vi "Update montage.vi"(4 "Frames info":T1, 6 "Frame's rel. index":i32=1 min=0, 8 "Error in":errorcluster, 9 "Single patch image":T2, 10 "Coordinates of montage positions":cluster{"Offset Left/Top":i32[]}[](array[cluster]), 11 "Image (Montage)":T2) -> (0 "error out":errorcluster, 3 "Image (Montage)":T2)   [LabVIEW 2020]
uses:
  <vilib>/vision/Image Controls.llb/IMAQ Image.ctl
  <vilib>/vision/NI_Vision_Development_Module.lvlib
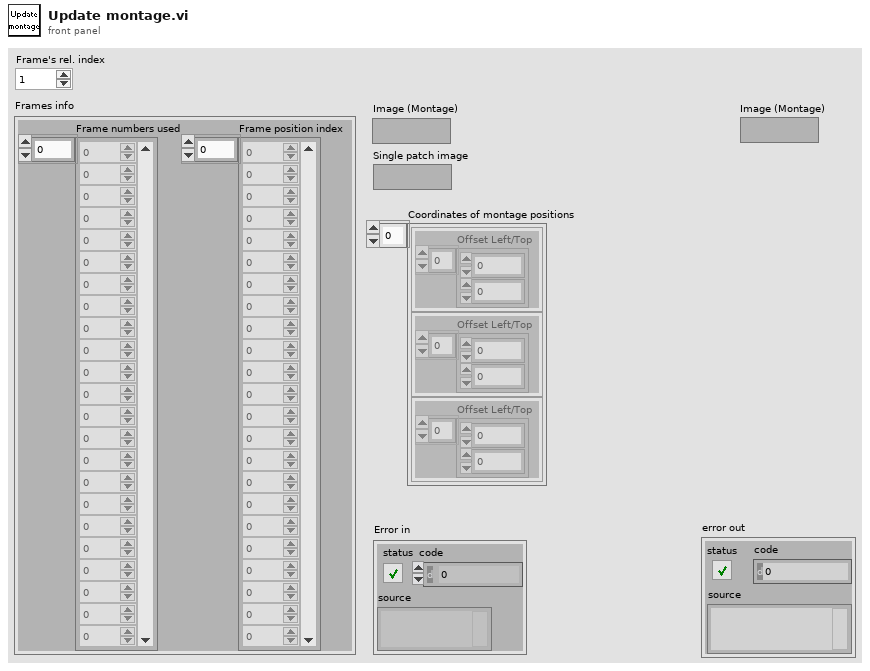
[diagram p1: front panel]
types:
  T1 = cluster{"Frame numbers used":i32[], "Frame position index":i32[]}
  T2 = typedef "IMAQ Image.ctl" = refnum<image>
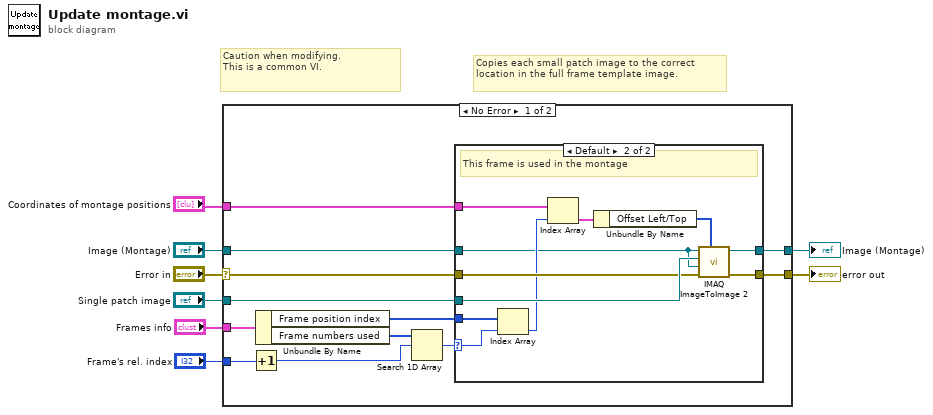
[diagram p0: block diagram]
diagram:
  # "Caution when modifying.\nThis is a common VI."
  # "Copies each small patch image to the correct location in the full frame template image."
  n1 = case shown="No Error" "Error in" {
    selector: "Error in" -> [w9 w35]
    tunnel: [w20 w34] -> w8
    tunnel: [w19 w35] -> w7
    tunnel: "Single patch image" -> [w18 _]
    tunnel: "Image (Montage)" -> [w17 w34]
    tunnel: "Coordinates of montage positions" -> [w16 _]
    tunnel: "Frames info" -> [w15 _]
    tunnel: "Frame's rel. index" -> [w14 _]
    frame No Error {
      n2 = Increment(x=w14) -> (x+1=w12:i32)
      n3 = Unbundle By Name(w15) -> ("Frame position index"=w11:i32[], "Frame numbers used"=w13:i32[])
      n4 = Search 1D Array(1D array=w13, element=w12) -> (index of element=w10:i32)  [unwired: 1 in]
      n5 = case shown="Default" w10 {
        selector: w10 -> [_ w24]
        tunnel: [w22 w33] -> w20
        tunnel: [w21 w31] -> w19
        tunnel: w18 -> [_ w30]
        tunnel: w17 -> [w22 w23]
        tunnel: w9 -> [w21 w29]
        tunnel: w16 -> [_ w28]
        tunnel: w11 -> [_ w26]
        frame -1 {
          # "This frame is not used in the montage"
        }
        frame Default {
          # "This frame is used in the montage"
          n6 = Index Array(array=w26, index=w24) -> (element=w25:i32)
          n7 = Index Array(array=w28, index=w25) -> (element=w27:cluster{"Offset Left/Top":i32[]})
          n8 = Unbundle By Name(w27) -> ("Offset Left/Top"=w32:i32[])
          n9 = call "IMAQ ImageToImage 2"("Offset Left/Top"=w32, "error in (no error)"=w29, "Image Dst"=w23, "Image Src (Small)"=w30, "Image Src (Large)"=w23) -> ("error out"=w31:errorcluster, "Image Dst Out"=w33:T2)  [unwired: 1 in, 4 out]
        }
      }
    }
    frame Error {
    }
  }
  "Image (Montage)" <- w8
  "error out" <- w7
